vi "HoldData_FGV.vi"(7 "HoldData_mods":T1, 8 "error in":errorcluster, 11 "DataIn":variant) -> (0 "error out":errorcluster, 3 "DataOut":variant)   [LabVIEW 2017]
uses:
  HoldData_mods.ctl
  HoldData_data.ctl
  DataForColision.ctl
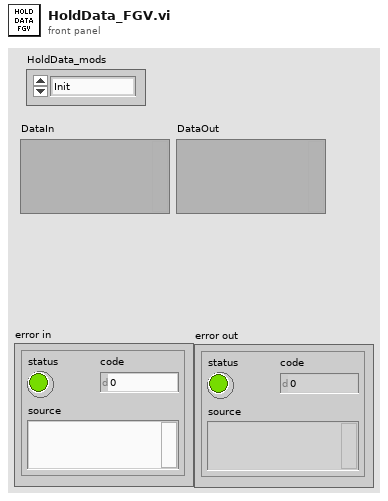
[diagram p1: front panel]
types:
  T1 = typedef "HoldData_mods.ctl" = enum16{"Init", "NewAster", "UpdateAster", "RemoveAster", "GetAsterData", "NewShoot", "UpdateShoot", "RemoveShoot", "GetShootData", "End"}
  T2 = typedef "HoldData_data.ctl" = cluster{"ShootData":T3[], "AsterData":T3[]}
  T3 = typedef "DataForColision.ctl" = cluster{"X":dbl, "Y":dbl, "Size":dbl, "ID":i32}
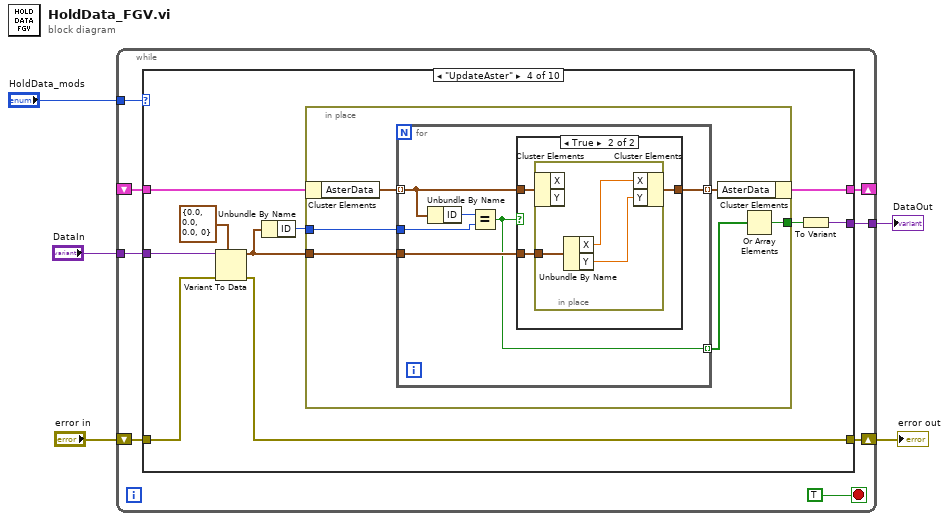
[diagram p0: block diagram]
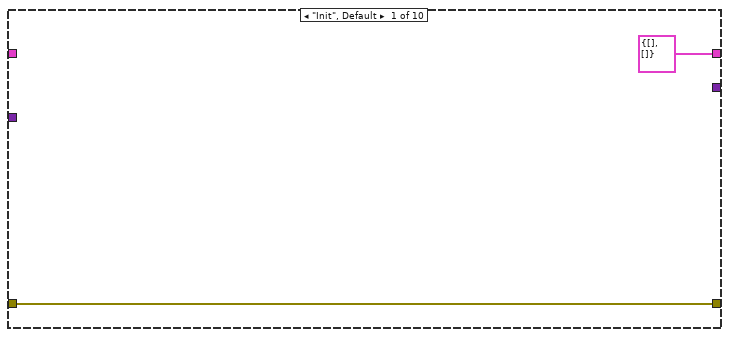
[diagram p2: hidden frame]
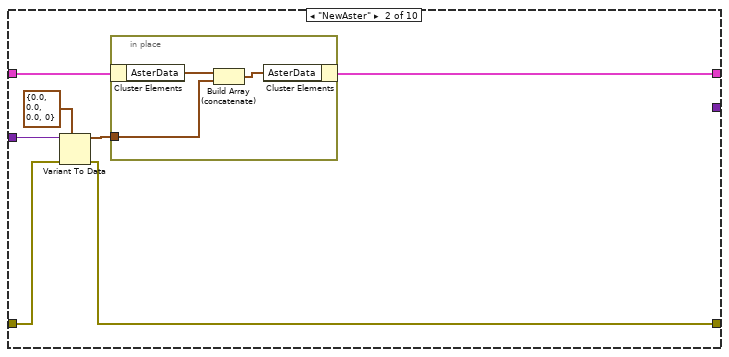
[diagram p3: hidden frame]
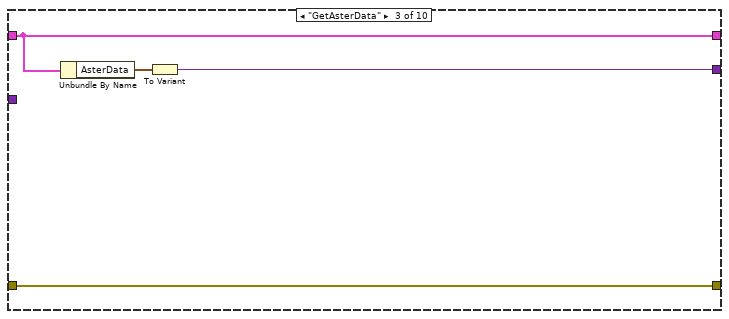
[diagram p4: hidden frame]
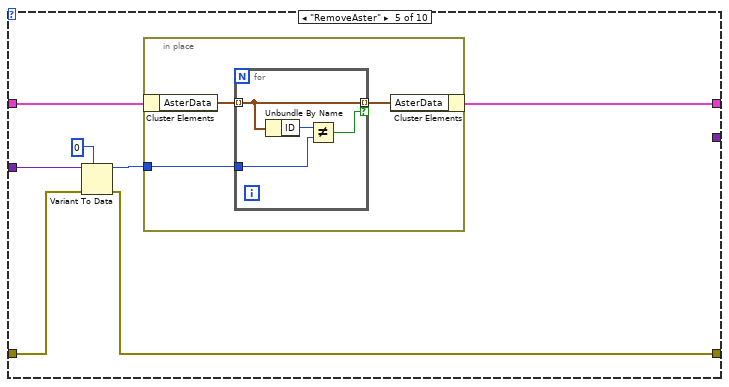
[diagram p6: hidden frame]
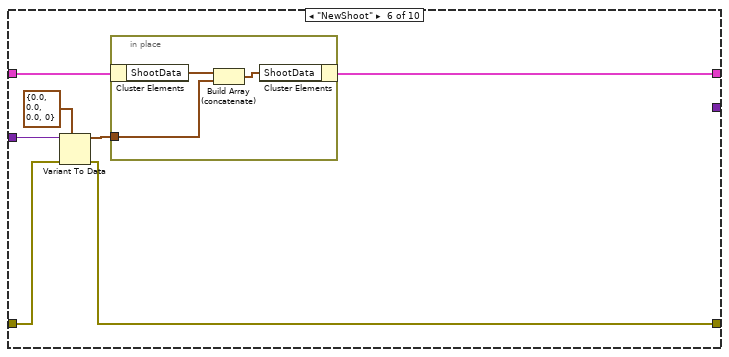
[diagram p7: hidden frame]
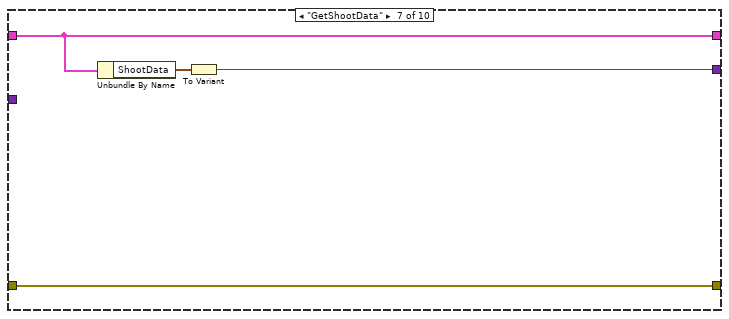
[diagram p8: hidden frame]
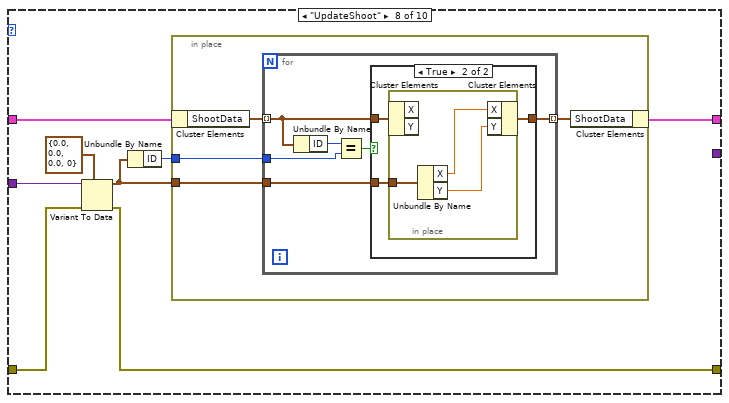
[diagram p9: hidden frame]
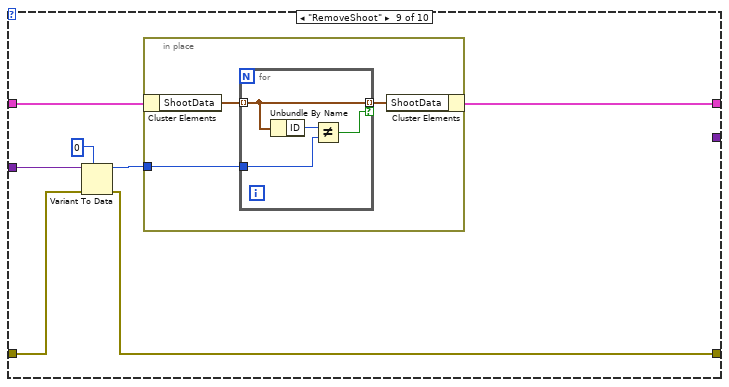
[diagram p11: hidden frame]
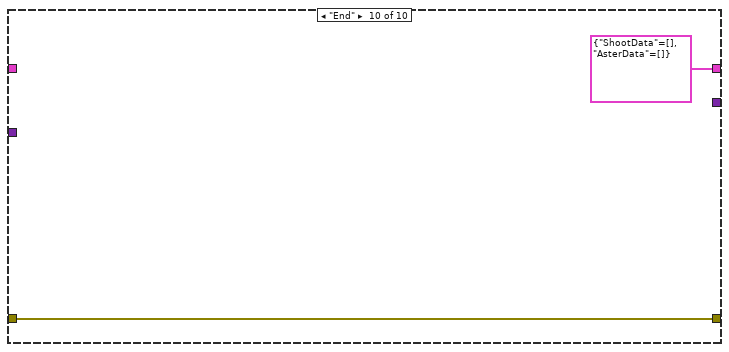
[diagram p12: hidden frame]
diagram:
  n1 = while {
    shift-right: [w9] -> w4
    shift-left: "error in" -> [w13]
    tunnel: "DataIn" -> [w11]
    tunnel: "HoldData_mods" -> [w10]
    shift-right: [w8] -> _
    shift-left: _ -> [w7]
    tunnel: [w6] -> w1
    stop <- TRUE stop-if-true
    n2 = case shown="\"UpdateAster\"" w10 {
      tunnel: w13 -> [w15 w21 w26 w37 w64 w78 w83 w92 w117 w127]
      tunnel: w11 -> [_ w22 _ w38 w65 w79 _ w93 w118 _]
      tunnel: [w15 w17 w26 w35 w62 w74 w83 w90 w115 w127] -> w9
      tunnel: [T2 {"ShootData"=[], "AsterData"=[]} ("HoldData_data") w16 w29 w33 w61 w73 w85 w88 w114 T2 {"ShootData"=[], "AsterData"=[]} ("HoldData_data")] -> w8
      tunnel: w7 -> [_ w19 w29 w36 w63 w76 w85 w91 w116 _]
      tunnel: [_ _ w27 w30 _ _ w84 _ _ _] -> w6
      frame "Init", Default {
      }
      frame "NewAster" {
        n3 = Variant To Data(error in=w21, type=T3 {"X"=0.0, "Y"=0.0, "Size"=0.0, "ID"=0} ("DataForColision"), Variant=w22) -> (data=w18:T3, error out=w17:errorcluster)
        n4 = in-place {
          in-place-border: w18 -> [w24]
          n5 = in-place-cluster #1(w19) -> ("AsterData"=w25:T3[])
          n6 = Build Array (concatenate)(w25, w24) -> (w23:T3[])
          n7 = in-place-cluster #1("AsterData"=w23) -> (w16:T2)
        }
      }
      frame "GetAsterData" {
        n8 = Unbundle By Name(w29) -> ("AsterData"=w28:T3[])
        n9 = To Variant(anything=w28) -> (Variant=w27:variant)
      }
      frame "UpdateAster" {
        n10 = Variant To Data(error in=w37, type=T3 {"X"=0.0, "Y"=0.0, "Size"=0.0, "ID"=0} ("DataForColision"), Variant=w38) -> (data=w32:T3, error out=w35:errorcluster)
        n11 = Unbundle By Name(w32) -> ("ID"=w34:i32)
        n12 = in-place {
          in-place-border: w34 -> [w44]
          in-place-border: w32 -> [w42]
          in-place-border: [w40] -> w31
          n13 = in-place-cluster #2(w36) -> ("AsterData"=w45:T3[])
          n14 = for {
            tunnel: w45 -> [w51] mode=indexing
            tunnel: w44 -> [w49]
            tunnel: [w48] -> w43 mode=indexing
            tunnel: w42 -> [w47]
            tunnel: [w46] -> w41 mode=indexing
            n15 = Unbundle By Name(w51) -> ("ID"=w50:i32)
            n16 = Equal?(x=w50, y=w49) -> (x = y?=w46:bool)
            n17 = case shown="True" w46 {
              tunnel: w51 -> [w52 w55]
              tunnel: [w52 w54] -> w48
              tunnel: w47 -> [_ w53]
              frame False {
              }
              frame True {
                n18 = in-place {
                  in-place-border: w53 -> [w58]
                  n19 = in-place-cluster #3(w55) -> ()  [unwired: 2 out]
                  n20 = Unbundle By Name(w58) -> ("X"=w57:dbl, "Y"=w56:dbl)
                  n21 = in-place-cluster #3("X"=w57, "Y"=w56) -> (w54:T3)
                }
              }
            }
          }
          n22 = in-place-cluster #2("AsterData"=w43) -> (w33:T2)
          n23 = Or Array Elements(Boolean array=w41) -> (logical OR=w40:bool)
        }
        n24 = To Variant(anything=w31) -> (Variant=w30:variant)
      }
      frame "RemoveAster" {
        n25 = Variant To Data(error in=w64, type=0, Variant=w65) -> (data=w59:i32, error out=w62:errorcluster)
        n26 = in-place {
          in-place-border: w59 -> [w67]
          n27 = in-place-cluster #4(w63) -> ("AsterData"=w68:T3[])
          n28 = for {
            tunnel: w68 -> [w69] mode=indexing
            tunnel: w67 -> [w71]
            tunnel: [w69] -> w66 mode=indexing if=w70
            n29 = Unbundle By Name(w69) -> ("ID"=w72:i32)
            n30 = Not Equal?(x=w72, y=w71) -> (x != y?=w70:bool)
          }
          n31 = in-place-cluster #4("AsterData"=w66) -> (w61:T2)
        }
      }
      frame "NewShoot" {
        n32 = Variant To Data(error in=w78, type=T3 {"X"=0.0, "Y"=0.0, "Size"=0.0, "ID"=0} ("DataForColision"), Variant=w79) -> (data=w75:T3, error out=w74:errorcluster)
        n33 = in-place {
          in-place-border: w75 -> [w81]
          n34 = in-place-cluster #5(w76) -> ("ShootData"=w82:T3[])
          n35 = Build Array (concatenate)(w82, w81) -> (w80:T3[])
          n36 = in-place-cluster #5("ShootData"=w80) -> (w73:T2)
        }
      }
      frame "GetShootData" {
        n37 = Unbundle By Name(w85) -> ("ShootData"=w86:T3[])
        n38 = To Variant(anything=w86) -> (Variant=w84:variant)
      }
      frame "UpdateShoot" {
        n39 = Variant To Data(error in=w92, type=T3 {"X"=0.0, "Y"=0.0, "Size"=0.0, "ID"=0} ("DataForColision"), Variant=w93) -> (data=w87:T3, error out=w90:errorcluster)
        n40 = Unbundle By Name(w87) -> ("ID"=w89:i32)
        n41 = in-place {
          in-place-border: w89 -> [w97]
          in-place-border: w87 -> [w95]
          n42 = in-place-cluster #6(w91) -> ("ShootData"=w98:T3[])
          n43 = for {
            tunnel: w98 -> [w104] mode=indexing
            tunnel: w97 -> [w102]
            tunnel: [w101] -> w96 mode=indexing
            tunnel: w95 -> [w99]
            n44 = Unbundle By Name(w104) -> ("ID"=w103:i32)
            n45 = Equal?(x=w103, y=w102) -> (x = y?=w100:bool)
            n46 = case shown="True" w100 {
              tunnel: w104 -> [w105 w108]
              tunnel: [w105 w107] -> w101
              tunnel: w99 -> [_ w106]
              frame False {
              }
              frame True {
                n47 = in-place {
                  in-place-border: w106 -> [w111]
                  n48 = in-place-cluster #7(w108) -> ()  [unwired: 2 out]
                  n49 = Unbundle By Name(w111) -> ("X"=w110:dbl, "Y"=w109:dbl)
                  n50 = in-place-cluster #7("X"=w110, "Y"=w109) -> (w107:T3)
                }
              }
            }
          }
          n51 = in-place-cluster #6("ShootData"=w96) -> (w88:T2)
        }
      }
      frame "RemoveShoot" {
        n52 = Variant To Data(error in=w117, type=0, Variant=w118) -> (data=w112:i32, error out=w115:errorcluster)
        n53 = in-place {
          in-place-border: w112 -> [w120]
          n54 = in-place-cluster #8(w116) -> ("ShootData"=w121:T3[])
          n55 = for {
            tunnel: w121 -> [w122] mode=indexing
            tunnel: w120 -> [w124]
            tunnel: [w122] -> w119 mode=indexing if=w123
            n56 = Unbundle By Name(w122) -> ("ID"=w125:i32)
            n57 = Not Equal?(x=w125, y=w124) -> (x != y?=w123:bool)
          }
          n58 = in-place-cluster #8("ShootData"=w119) -> (w114:T2)
        }
      }
      frame "End" {
      }
    }
  }
  "error out" <- w4
  "DataOut" <- w1
